vi "Deserialize.vi"(8 "error in (no error)":errorcluster, 10 "Serialized PE Spec":string, 11 "RandomNumberGenerator Controller in":refnum<class "RandomNumberGenerator Controller.lvclass">) -> (0 "error out":errorcluster, 3 "RandomNumberGenerator Controller out":refnum<class "RandomNumberGenerator Controller.lvclass">)   [LabVIEW 2020, in "RandomNumberGenerator.lvlib" / "RandomNumberGenerator Controller.lvclass"]
doc: "<b>Deserailize</b>\nThis VI loads the configuration that has been deserialized into the plugin controller object."
uses:
  RandomNumberGenerator Controller.lvclass
  RandomNumberGenerator Controller.lvclass/RandomNumberGenerator Controller.ctl
  PE/Get Configuration Version.vi
  PE/Mutate Configuration to Current.vi
  PE/Default Configuration Parameters.vi
  <vilib>/ADAS Record/Utilities/Config/Data Converter/Populate Container from JSON.vi
  PE/RandomNumberGenerator.lvclass
panel:
  # "#via_ignore"
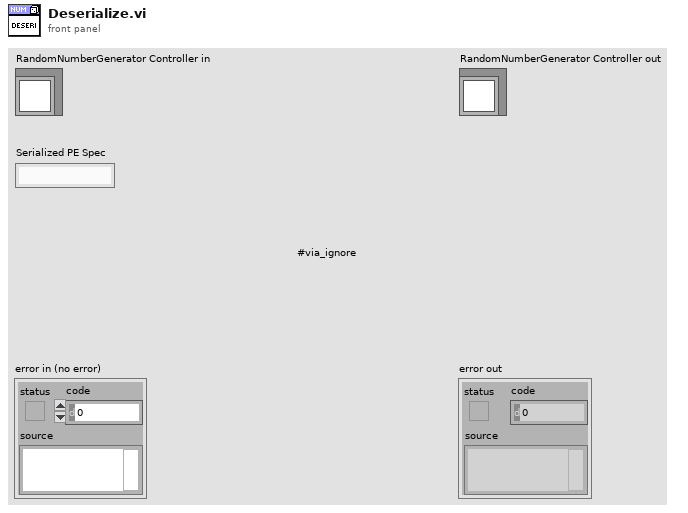
[diagram p1: front panel]
types:
  T1 = typedef "RandomNumberGenerator.lvlib/RandomNumberGenerator.lvclass/Configuration.ctl" = cluster{"Parameter1":string}
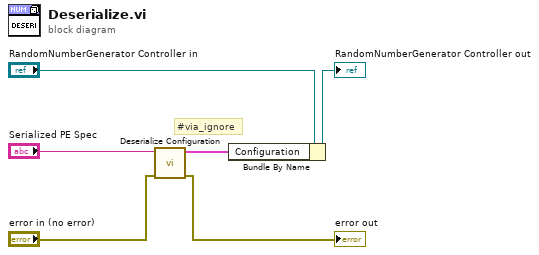
[diagram p0: block diagram]
diagram:
  # "#via_ignore"
  n1 = call "Deserialize Configuration.vi"("error in (no error)"="error in (no error)", "Serialized Configuration"="Serialized PE Spec") -> ("error out"=→"error out":errorcluster, "Configuration"=w3:T1)  [unwired: 8 in]
  n2 = Bundle By Name(cluster="RandomNumberGenerator Controller in", "Configuration"=w3) -> (→"RandomNumberGenerator Controller out":refnum<class "RandomNumberGenerator Controller.lvclass">)
